vi "Create.vi"(8 "Error In":errorcluster, 10 "Package Suffix":string="CE", 11 "Package Path":path) -> (0 "Error Out":errorcluster)   [LabVIEW 2019, in "CEPM.lvlib"]
uses:
  CEPM.lvlib
  <vilib>/National Instruments/NIPM API (Beta)/NIPM_API.lvlib
  <vilib>/SLL Toolkit/SLL File IO/SLL File IO.lvlib
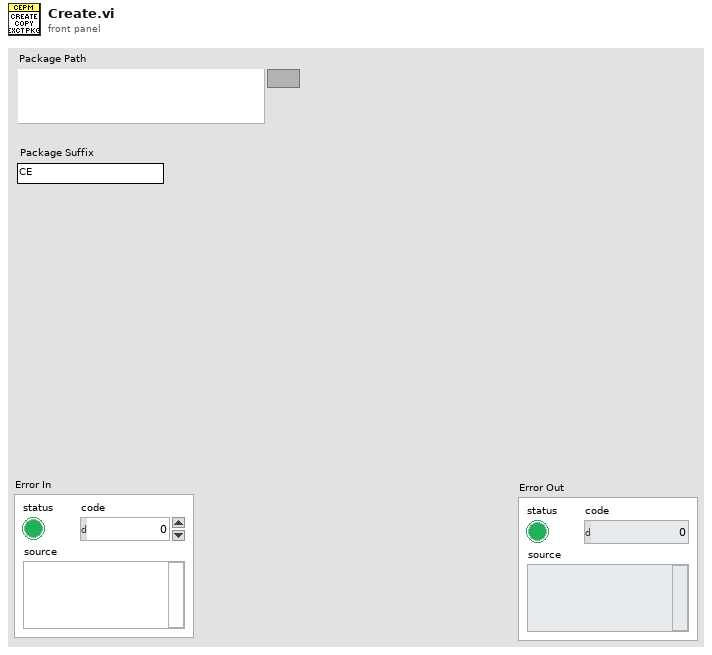
[diagram p1: front panel]
types:
  T1 = typedef "NIPM_API.lvlib/package attributes.ctl" = cluster{"Package Name":string, "Display name":string, "Version":string, "Display version":string, "Synopsis":string, "Description":string, "Maintainer":string, "Maintainer email address":string, "Category":string, "Homepage":string, "Release notes":string, "Depends":string[], "Recommends":string[], "Suggests":string[], "Conflicts":string[], "Provides":string[], "Replaces":string[], "Supplements":string[], "Enhances":string[], "Product":bool, "User visible":bool, "Installed size (KB)":u64, "Package filesize (bytes)":u64, "Architecture":string, "Agent":string, "MD5Checksum":string}
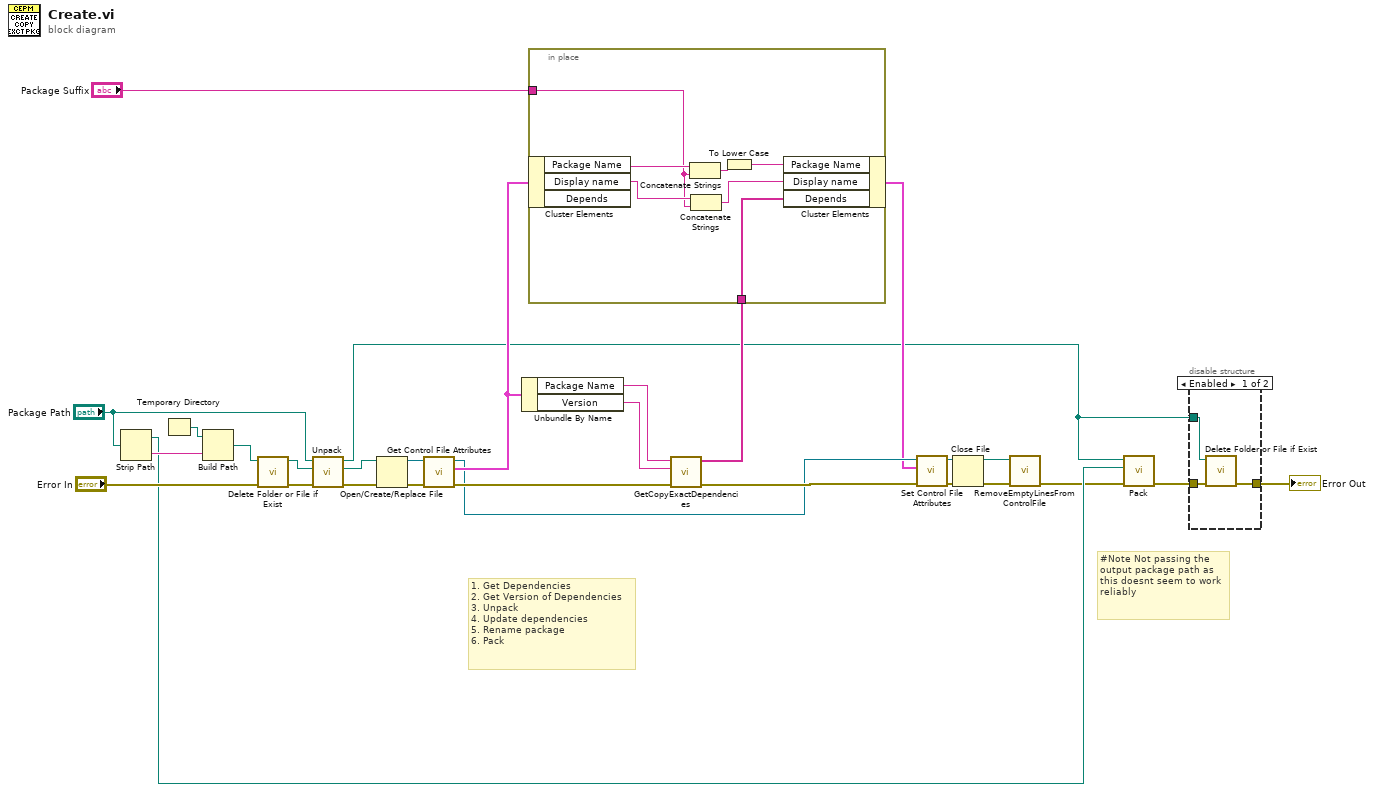
[diagram p0: block diagram]
diagram:
  # "#Note Not passing the output package path as this doesnt seem to work reliably"
  # "1. Get Dependencies\n2. Get Version of Dependencies\n3. Unpack\n4. Update dependencies\n5. Rename package\n6. Pack"
  n1 = Strip Path(path="Package Path") -> (stripped path=w8:path, name=w23:string)
  n2 = Temporary Directory() -> (w25:path)
  n3 = Build Path(base path=w25, name or relative path=w23) -> (appended path=w22:path)
  n4 = call <vilib>:"Delete Folder or File if Exist.vi"("error in (no error)"="Error In", "Path"=w22) -> ("error out"=w20:errorcluster, "Path out"=w21:path)  [unwired: 8 in]
  n5 = call <vilib>:"Unpack.vi"("error in"=w20, "destination folder"=w21, "nipkg filepath"="Package Path") -> ("error out"=w26:errorcluster, "control filepath"=w27:path, "unpacked folderpath"=w2:path)  [unwired: 4 in, 2 out]
  n6 = Open/Create/Replace File(file path (use dialog)=w27, error in=w26) -> (refnum out=w28:refnum<file>, error out=w29:errorcluster)  [unwired: 4 in, 1 out]
  n7 = call <vilib>:"Get Control File Attributes.vi"("error in (no error)"=w29, "control file refnum in"=w28) -> ("error out"=w17:errorcluster, "package attributes"=w14:T1, "control file refnum out"=w10:refnum<file>)  [unwired: 7 in]
  n8 = Unbundle By Name(w14) -> ("Package Name"=w18:string, "Version"=w15:string)
  n9 = call "GetCopyExactDependencies.vi"("Error In"=w17, "Package Version"=w15, "Package Name"=w18) -> ("Error Out"=w16:errorcluster, "Copy Exact Dependencies"=w12:string[])  [unwired: 7 in]
  n10 = in-place {
    in-place-border: "Package Suffix" -> [w33]
    in-place-border: w12 -> [w30]
    n11 = in-place-cluster #1(w14) -> ("Package Name"=w36:string, "Display name"=w34:string)  [unwired: 1 out]
    n12 = Concatenate Strings(w36, w33) -> (w35:string)
    n13 = Concatenate Strings(w34, w33) -> (w32:string)
    n14 = To Lower Case(string=w35) -> (all lower case string=w31:string)
    n15 = in-place-cluster #1("Package Name"=w31, "Display name"=w32, "Depends"=w30) -> (w9:T1)
  }
  n16 = call <vilib>:"Set Control File Attributes.vi"("error in (no error)"=w16, "package attributes"=w9, "control file refnum in"=w10) -> ("error out"=w11:errorcluster, "control file refnum out"=w7:refnum<file>)  [unwired: 7 in]
  n17 = Close File(refnum=w7, error in=w11) -> (path=w4:path, error out=w6:errorcluster)
  n18 = call "RemoveEmptyLinesFromControlFile.vi"("Error In"=w6, "Control File Path"=w4) -> ("Error Out"=w5:errorcluster)  [unwired: 9 in]
  n19 = call <vilib>:"Pack.vi"("error in"=w5, "destination folder"=w8, "source folder"=w2) -> ("error out"=w3:errorcluster)  [unwired: 7 in, 1 out]
  n20 = disable-structure shown="Enabled" {
    disable-tunnel: w3 -> [w39 w40]
    disable-tunnel: w2 -> [w38 _]
    disable-tunnel: [w37 w40] -> w1
    frame Enabled {
      n21 = call <vilib>:"Delete Folder or File if Exist.vi"("error in (no error)"=w39, "Path"=w38) -> ("error out"=w37:errorcluster)  [unwired: 8 in, 1 out]
    }
    frame Disabled {
    }
  }
  "Error Out" <- w1
